vi "No Op.vi"() -> (2 "Msg":refnum<class "Msg.lvclass">)   [LabVIEW 2020, in "jettl.lvlib" / "No Op Msg.lvlib"]
uses:
  No Op Msg.lvlib
  Msg/Msg.lvclass
  No Op Msg/No Op Msg.lvclass
  C:/git/jettl/src/jettl/jettl/Msg/Msg.lvclass
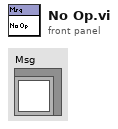
[diagram p1: front panel]
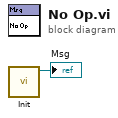
[diagram p0: block diagram]
diagram:
  n1 = call "Init.vi"() -> ("No Op Msg out"=→"Msg":refnum<class "No Op Msg.lvclass">)  [unwired: 11 in]
